vi "ReadConfig.vi"(4 "error in":errorcluster, 7 "section":string) -> (0 "error out":errorcluster, 2 "key":string[](array[string]), 3 "value":string[](array[string]))   [LabVIEW 2015]
uses:
  <vilib>/Utility/config.llb/Read Key (String).vi
  <vilib>/Utility/config.llb/NI_LVConfig.lvlib
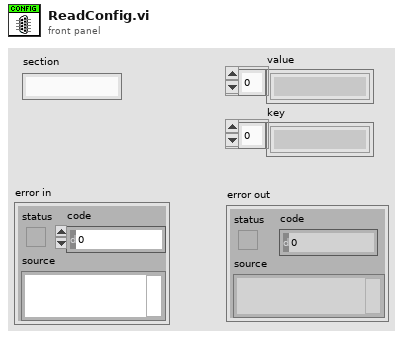
[diagram p1: front panel]
types:
  T1 = typedef "NI_LVConfig.lvlib/Config Data RefNum.ctl" = refnum<k1>
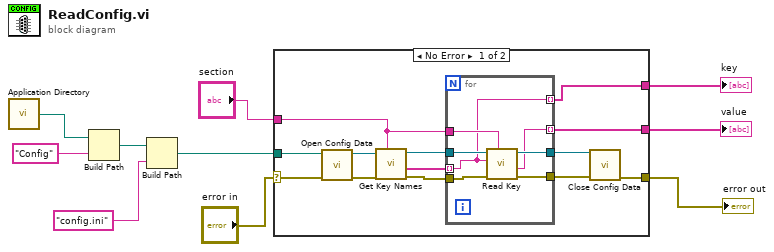
[diagram p0: block diagram]
diagram:
  n1 = call <vilib>:"Application Directory.vi"() -> ("Application Directory"=w1:path)
  n2 = Build Path(base path=w1, name or relative path="Config") -> (appended path=w5:path)
  n3 = Build Path(base path=w5, name or relative path="config.ini" ("config File")) -> (appended path=w8:path)
  n4 = case shown="No Error" "error in" {
    selector: "error in" -> [w13 w31]
    tunnel: w8 -> [w23 _]
    tunnel: "section" -> [w17 _]
    tunnel: [w14 w31] -> w6
    tunnel: [w12 _] -> w3
    tunnel: [w11 _] -> w2
    frame No Error {
      n5 = call <vilib>:"Open Config Data.vi"("error in (no error)"=w13, "configuration file path"=w23) -> ("error out"=w21:errorcluster, "refnum"=w22:T1)  [unwired: 7 in, 1 out]
      n6 = call <vilib>:"Get Key Names.vi"("section"=w17, "error in (no error)"=w21, "refnum"=w22) -> ("error out"=w18:errorcluster, "key names"=w20:string[], "refnum out"=w19:T1)  [unwired: 5 in, 1 out]
      n7 = for {
        tunnel: w20 -> [w25] mode=indexing
        tunnel: w19 -> [w30]
        tunnel: w18 -> [w29]
        tunnel: w17 -> [w28]
        tunnel: [w24] -> w11 mode=indexing
        tunnel: [w27] -> w16
        tunnel: [w26] -> w15
        tunnel: [w25] -> w12 mode=indexing
        n8 = call-poly <vilib>:"Read Key.vi"("section"=w28, "error in (no error)"=w29, "key"=w25, "refnum"=w30) -> ("error out"=w26:errorcluster, "value"=w24:string, "refnum out"=w27:T1)  [unwired: 4 in, 1 out]
      }
      n9 = call <vilib>:"Close Config Data.vi"("error in (no error)"=w15, "refnum"=w16) -> ("error out"=w14:errorcluster)  [unwired: 8 in, 1 out]
    }
    frame Error {
    }
  }
  "error out" <- w6
  "value" <- w2
  "key" <- w3
